vi "Asym Balance Square.vi"() -> ()   [LabVIEW 2018]
uses:
  <vilib>/measure/NI_MABase.lvlib
panel:
  out "Negative (Low)\nAmplitude":dbl
  out "Samples\nper Period":dbl
  in  "Duty Cycle (%)":u64
  in  "Positive (High)\nAmplitude":ext
  in  "Frequency (Hz)":u64
  out "Waveform Graph":waveform(dbl)(graph)
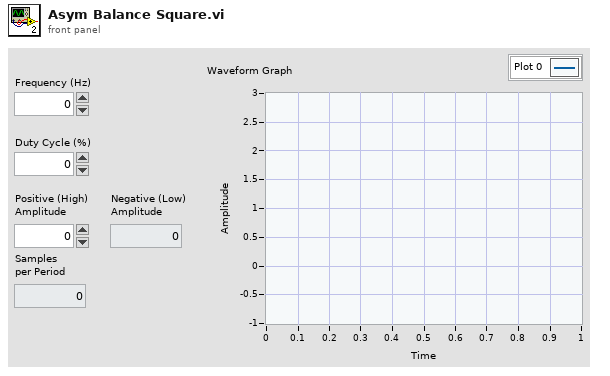
[diagram p1: front panel]
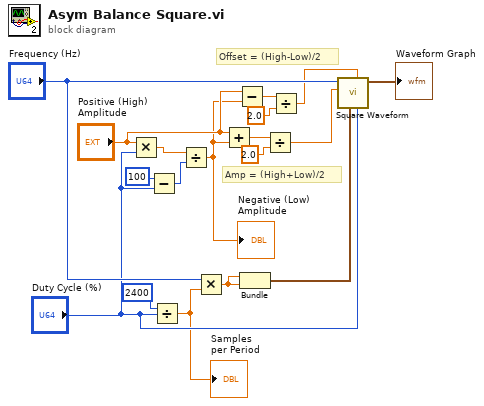
[diagram p0: block diagram]
diagram:
  # "Offset = (High-Low)/2"
  # "Amp = (High+Low)/2"
  n1 = Multiply(x="Positive (High)\nAmplitude", y="Duty Cycle (%)") -> (x*y=w10:ext)
  n2 = Subtract(x=u64 100, y="Duty Cycle (%)") -> (x-y=w11:u64)
  n3 = Divide(x=u64 2400, y="Duty Cycle (%)") -> (x/y=w2:dbl)
  "Samples\nper Period" <- w2
  n4 = Divide(x=w10, y=w11) -> (x/y=w1:ext)
  "Negative (Low)\nAmplitude" <- w1
  n5 = Multiply(x="Frequency (Hz)", y=w2) -> (x*y=w15:dbl)
  n6 = Add(x="Positive (High)\nAmplitude", y=w1) -> (x+y=w8:ext)
  n7 = Subtract(x="Positive (High)\nAmplitude", y=w1) -> (x-y=w4:ext)
  n8 = Bundle(w15, w15) -> (w18:cluster{dbl, dbl})  [unwired: 1 in]
  n9 = Divide(x=w8, y=2.0) -> (x/y=w7:ext)
  n10 = Divide(x=w4, y=2.0) -> (x/y=w3:ext)
  n11 = call <vilib>:"Square Waveform.vi"("duty cycle (%)"="Duty Cycle (%)", "offset"=w3, "sampling info"=w18, "amplitude"=w7, "frequency"="Frequency (Hz)") -> ("signal out"=→"Waveform Graph":waveform(dbl))  [unwired: 5 in, 1 out]
